vi "base64 encode.vi"(1 "data":u8[](array[numeric]) format="%.0x") -> (0 "base64 encoded string":string)   [LabVIEW 2019, in "WebSocket Server Toolkit.lvlib"]
uses:
  WebSocket Server Toolkit.lvlib
  binary to char.ctl
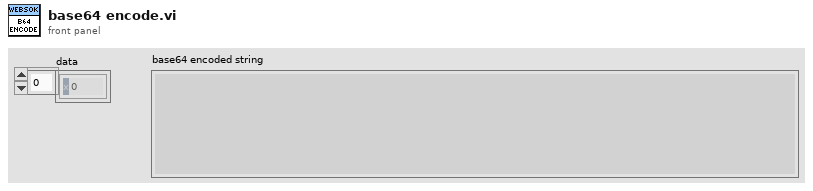
[diagram p1: front panel]
types:
  T1 = typedef "WebSocket Server Toolkit.lvlib/binary to char.ctl" = map{u8, u8}
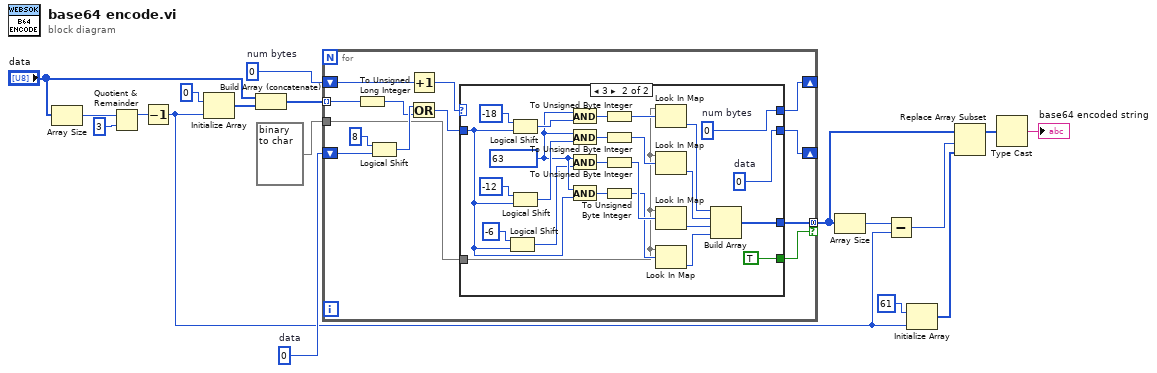
[diagram p0: block diagram]
diagram:
  w9 = u32 0  # data
  w10 = u32 0  # num bytes
  n1 = Array Size(array="data") -> (size(s)=w18:i32)
  n2 = Quotient & Remainder(x=w18, y=3) -> (x-y*floor(x/y)=w13:i32)  [unwired: 1 out]
  n3 = Decrement(x=w13) -> (x-1=w2:i32)
  n4 = Initialize Array(u8 0, w2) -> (w15:u8[])
  n5 = Build Array (concatenate)("data", w15) -> (w12:u8[])
  n6 = for {
    tunnel: w12 -> [w20] mode=indexing
    shift-right: [w24] -> _
    shift-left: w9 -> [w31]
    shift-right: [w25] -> _
    shift-left: w10 -> [w30]
    tunnel: T1 {0=65, 1=66, 2=67, 3=68, 4=69, 5=70, 6=71, 7=72, 8=73, 9=74, 10=75, 11=76, 12=77, 13=78, 14=79, 15=80, 16=81, 17=82, 18=83, 19=84, 20=85, 21=86, 22=87, 23=88, 24=89, 25=90, 26=97, 27=98, 28=99, 29=100, 30=101, 31=102, 32=103, 33=104, 34=105, 35=106, 36=107, 37=108, 38=109, 39=110, 40=111, 41=112, 42=113, 43=114, 44=115, 45=116, 46=117, 47=118, 48=119, 49=120, 50=121, 51=122, 52=48, 53=49, 54=50, 55=51, 56=52, 57=53, 58=54, 59=55, 60=56, 61=57, 62=43, 63=47} ("binary to char") -> [w19]
    tunnel: [w27] -> w3 mode=concatenating if=w26
    n7 = To Unsigned Long Integer(number=w20) -> (unsigned 32bit integer=w21:u32)
    n8 = Logical Shift(y=i16 8, x=w31) -> (x << y=w22:u32)
    n9 = Increment(x=w30) -> (x+1=w29:u32)
    n10 = Or(x=w22, y=w21) -> (x .or. y?=w28:u32)
    n11 = case shown="3" w29 {
      selector: w29 -> [w33 _]
      tunnel: w28 -> [w32 w39]
      tunnel: [_ w34] -> w27
      tunnel: [_ TRUE] -> w26
      tunnel: [w33 w57] -> w25
      tunnel: [w32 w56] -> w24
      tunnel: w19 -> [_ w40]
      frame Default {
      }
      frame 3 {
        w45 = u32 63 ("hi")
        w56 = u32 0  # data
        w57 = u32 0  # num bytes
        n12 = Logical Shift(y=i16 -6, x=w39) -> (x << y=w44:u32)
        n13 = Logical Shift(y=i16 -18, x=w39) -> (x << y=w52:u32)
        n14 = Logical Shift(y=i16 -12, x=w39) -> (x << y=w54:u32)
        n15 = And(x=w45, y=w52) -> (x .and. y?=w47:u32)
        n16 = And(x=w45, y=w54) -> (x .and. y?=w49:u32)
        n17 = And(x=w45, y=w44) -> (x .and. y?=w43:u32)
        n18 = And(x=w45, y=w39) -> (x .and. y?=w51:u32)
        n19 = To Unsigned Byte Integer(number=w47) -> (unsigned 8bit integer=w48:u8)
        n20 = To Unsigned Byte Integer(number=w49) -> (unsigned 8bit integer=w50:u8)
        n21 = To Unsigned Byte Integer(number=w43) -> (unsigned 8bit integer=w42:u8)
        n22 = To Unsigned Byte Integer(number=w51) -> (unsigned 8bit integer=w41:u8)
        n23 = Look In Map(map=w40, key=w48) -> (value=w38:u8)  [unwired: 1 in, 1 out]
        n24 = Look In Map(map=w40, key=w50) -> (value=w37:u8)  [unwired: 1 in, 1 out]
        n25 = Look In Map(map=w40, key=w42) -> (value=w36:u8)  [unwired: 1 in, 1 out]
        n26 = Look In Map(map=w40, key=w41) -> (value=w35:u8)  [unwired: 1 in, 1 out]
        n27 = Build Array(w38, w37, w36, w35) -> (w34:u8[])
      }
    }
  }
  n28 = Array Size(array=w3) -> (size(s)=w7:i32)
  n29 = Subtract(x=w7, y=w2) -> (x-y=w8:i32)
  n30 = Initialize Array(u8 61, w2) -> (w6:u8[])
  n31 = Replace Array Subset(array=w3, new element=w6, index=w8) -> (w5:u8[])
  n32 = Type Cast(x=w5) -> (*(type *) &x=→"base64 encoded string":string)  [unwired: 1 in]
